vi "Defaults.vi"(8 "error in (no error)":errorcluster, 11 "MB Slave in":refnum<class "MB Slave Simulator Base.lvclass">) -> (0 "error out":errorcluster, 3 "MB Slave out":refnum<class "MB Slave Simulator Base.lvclass">)   [LabVIEW 2021, in "MB Slave Simulator Base.lvclass"]
uses:
  MB Slave Simulator Base.lvclass
  <userlib>/S2 Labs/Module Framework/Modules/Modbus/Modbus Slave Base/Modbus Slave Base.lvclass
  MB Slave Simulator Base.lvclass/MB Slave Simulator Base.ctl
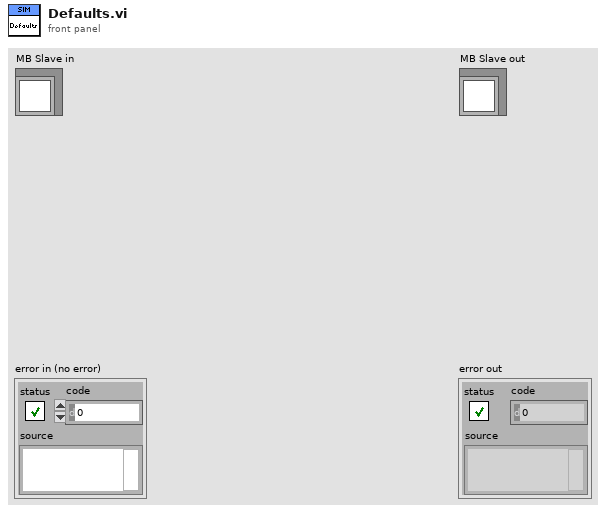
[diagram p1: front panel]
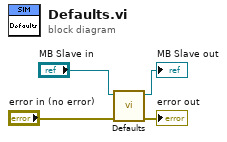
[diagram p0: block diagram]
diagram:
  n1 = call-parent "Defaults.vi"("error in (no error)"="error in (no error)", "MB Slave in"="MB Slave in") -> ("error out"=→"error out":errorcluster, "MB Slave out"=→"MB Slave out":refnum<class "MB Slave Simulator Base.lvclass">)  [unwired: 8 in]
